vi "Gen_2D_pattern.vi"(1 "Soften points":i32=3, 4 "Lissajous Cluster":cluster{"a":dbl, "b":dbl, "delta":dbl}={"a"=1.0, "b"=2.0, "delta"=0.0} {"delta" format="%_3g"; "b" format="%0.2p"; "a" format="%_3g"}, 5 "Home the stage after scan?":bool, 6 "Scan mode":T1(ring)=enum."Single Direction (Uniform)", 7 "Soften":bool, 8 "error in (no error)":errorcluster, 9 "asymmetry":dbl=0.9, 10 "Slow axis":T2, 11 "Fast axis":T2) -> (0 "error out":errorcluster, 2 "Waveform Graph":dbl[][](graph), 3 "Samples per channel":i32)   [LabVIEW 2014]
panel:
  in  "Pattern":T1(ring)=enum."Single Direction (Uniform)"
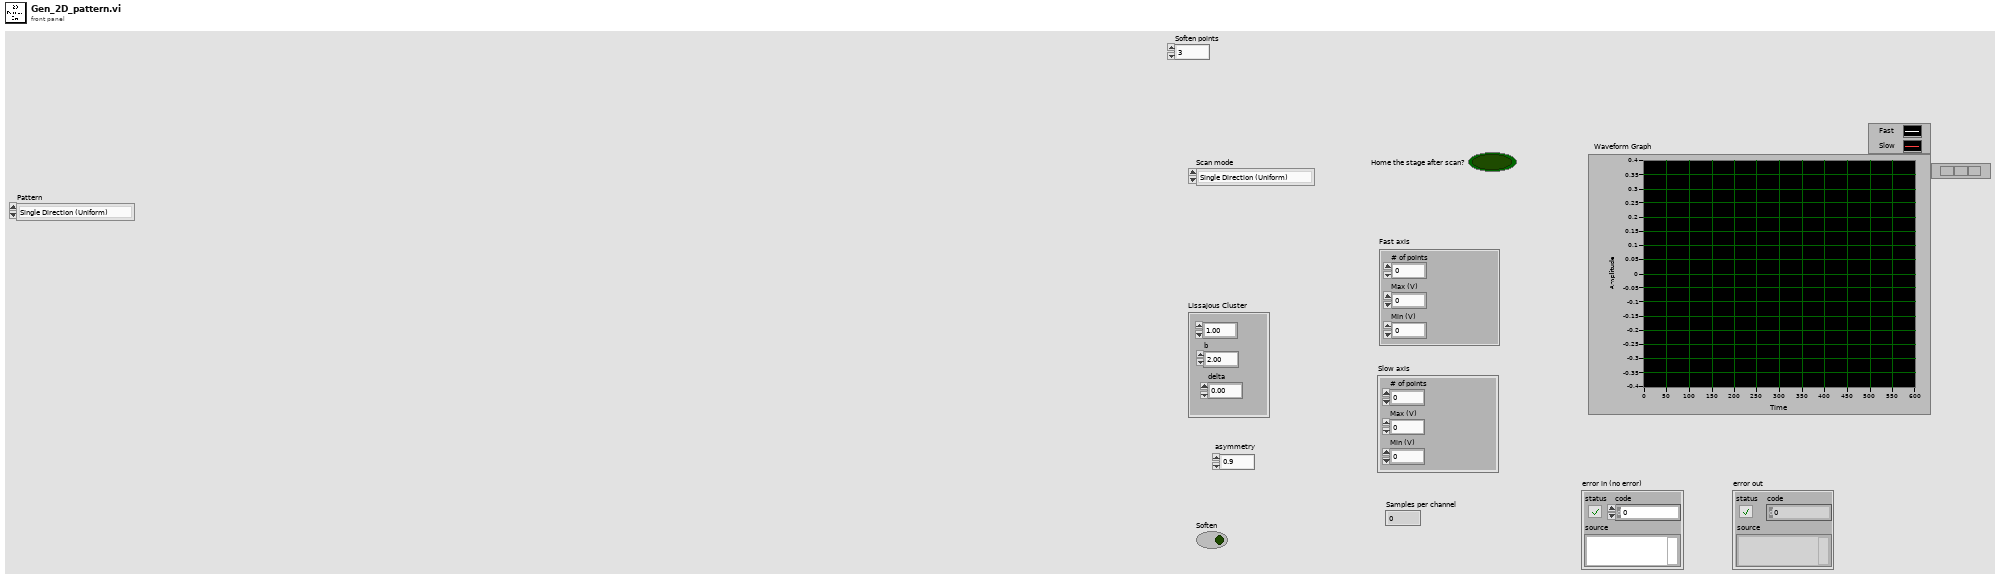
[diagram p1: front panel]
types:
  T1 = enum16{"Lissajous", "Adjustable sawtooth", "Single Direction (Uniform)", "Single Direction (Fast Reset)", "Bi-Directional"}
  T2 = cluster{"# of points":u16, "Max (V)":dbl, "Min (V)":dbl}
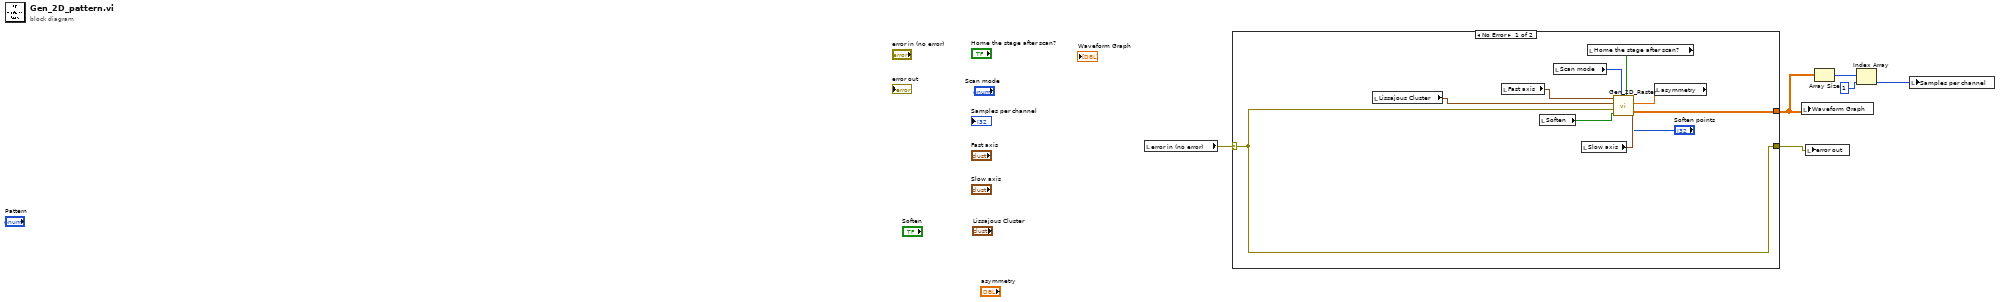
[diagram p0: block diagram]
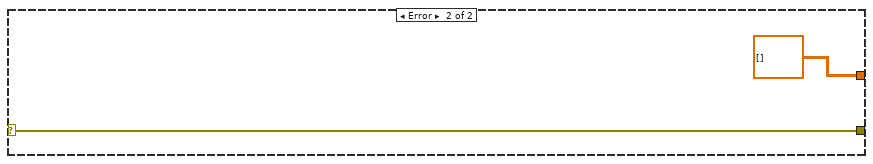
[diagram p2: hidden frame]
diagram:
  n1 = local read "error in (no error)"() -> (w6:errorcluster)
  n2 = case shown="No Error" w6 {
    selector: w6 -> [w9 w18]
    tunnel: [w9 w18] -> w5
    tunnel: [w16 dbl[][] []] -> w4
    frame No Error {
      n3 = local read "Lissajous Cluster"() -> (w11:cluster{"a":dbl, "b":dbl, "delta":dbl})
      n4 = local read "Fast axis"() -> (w14:T2)
      n5 = local read "Soften"() -> (w8:bool)
      n6 = local read "Scan mode"() -> (w13:T1)
      n7 = local read "Slow axis"() -> (w12:T2)
      n8 = local read "Home the stage after scan?"() -> (w15:bool)
      n9 = local read "asymmetry"() -> (w10:dbl)
      n10 = call "Gen_2D_Raster.vi"("Fast-axis Para"=w14, "Lissajous Cluster"=w11, "error in (no error)"=w9, "Soften"=w8, "Pattern"=w13, "Reset slow axis at End of Scan?"=w15, "asymmetry"=w10, "Soften points"="Soften points", "Slow-axis Para"=w12) -> ("2D Raster Pattern"=w16:dbl[][])  [unwired: 1 out]
    }
    frame Error {
    }
  }
  n11 = local write "Waveform Graph"(w4) -> ()
  n12 = local write "error out"(w5) -> ()
  n13 = Array Size(array=w4) -> (size(s)=w3:i32[])
  n14 = Index Array(array=w3, index=u8 1) -> (element=w1:i32)
  n15 = local write "Samples per channel"(w1) -> ()
